vi "Read Pre RTD.vi"(8 "error in":errorcluster, 11 "DAC RTD Temp in":refnum<class "DAC RTD Temp.lvclass">) -> (0 "error out":errorcluster, 3 "DAC RTD Temp out":refnum<class "DAC RTD Temp.lvclass">)   [LabVIEW 2019, in "DAC.lvlib" / "DAC RTD Temp.lvclass"]
uses:
  DAC RTD Temp.lvclass
  Results/Results Method.ctl
  Results/Heat Flow Results/Heat Flow Results.lvclass
  DAC RTD Temp.lvclass/DAC RTD Temp.ctl
  Results/Heat Flow Results/Heat Flow Results.lvclass/Heat Flow Results.ctl
  <vilib>/DAQmx/read.llb/DAQmx Read (Analog 1D DBL NChan 1Samp).vi
  <vilib>/DAQmx/miscellaneous.llb/DAQmx Fill In Error Info.vi
  Results/Results.lvlib
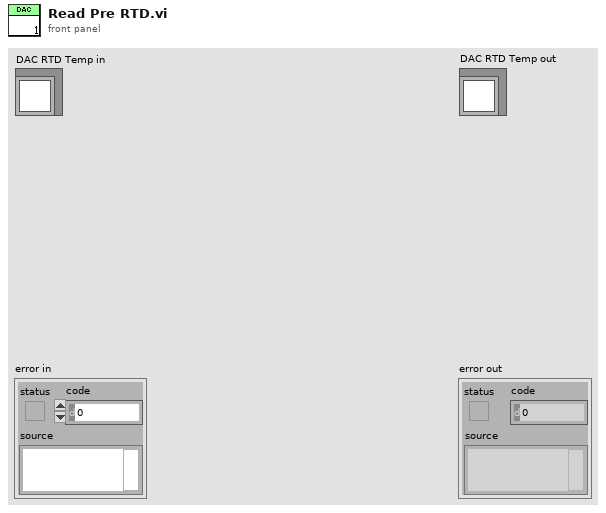
[diagram p1: front panel]
types:
  T1 = typedef "Results.lvlib/Results Method.ctl" = enum16{"Get", "Set"}
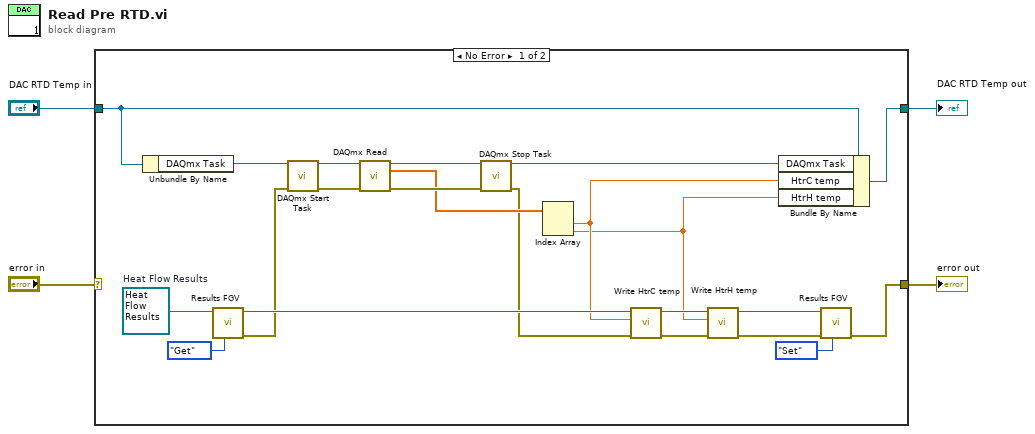
[diagram p0: block diagram]
diagram:
  n1 = case shown="No Error" "error in" {
    selector: "error in" -> [_ w28]
    tunnel: [w6 w28] -> w3
    tunnel: [w26 w27] -> w1
    tunnel: "DAC RTD Temp in" -> [w25 w27]
    frame No Error {
      w15 = refnum<class "Heat Flow Results.lvclass"> refnum  # Heat Flow Results
      n2 = Unbundle By Name(w25) -> ("DAQmx Task"=w24:refnum<k21>)
      n3 = call-dynamic "Results FGV.vi"("Method"=Results_Method."Get", "Results in"=w15) -> ("error out"=w5:errorcluster, "Results out"=w14:refnum<class "Heat Flow Results.lvclass">)  [unwired: 8 in]
      n4 = call <vilib>:"DAQmx Start Task.vi"("task/channels in"=w24, "error in"=w5) -> ("task out"=w23:refnum<k21>, "error out"=w20:errorcluster)  [unwired: 12 in]
      n5 = call-poly <vilib>:"DAQmx Read.vi"("task/channels in"=w23, "error in"=w20) -> ("task out"=w22:refnum<k21>, "data"=w18:dbl[], "error out"=w19:errorcluster)  [unwired: 11 in]
      n6 = call <vilib>:"DAQmx Stop Task.vi"("task/channels in"=w22, "error in"=w19) -> ("task out"=w21:refnum<k21>, "error out"=w9:errorcluster)  [unwired: 12 in]
      n7 = Index Array(array=w18) -> (element #1=w11:dbl, element #2=w10:dbl)  [unwired: 2 in]
      n8 = call "Write HtrC temp.vi"("error in (no error)"=w9, "HtrC temp"=w11, "Heat Flow Results in"=w14) -> ("error out"=w8:errorcluster, "Heat Flow Results out"=w13:refnum<class "Heat Flow Results.lvclass">)  [unwired: 7 in]
      n9 = call "Write HtrH temp.vi"("error in (no error)"=w8, "HtrH temp"=w10, "Heat Flow Results in"=w13) -> ("error out"=w7:errorcluster, "Heat Flow Results out"=w12:refnum<class "Heat Flow Results.lvclass">)  [unwired: 7 in]
      n10 = Bundle By Name(cluster=w25, "DAQmx Task"=w21, "HtrC temp"=w11, "HtrH temp"=w10) -> (w26:refnum<class "DAC RTD Temp.lvclass">)
      n11 = call-dynamic "Results FGV.vi"("Method"=Results_Method."Set", "error in"=w7, "Results in"=w12) -> ("error out"=w6:errorcluster)  [unwired: 7 in, 1 out]
    }
    frame Error {
    }
  }
  "error out" <- w3
  "DAC RTD Temp out" <- w1
